vi "72_Vision_RC Servo_DC_Moto_test_PID.vi"() -> ()   [LabVIEW 2018]
uses:
  <userlib>/KNR OS 4.0 LabVIEW Toolkit/Type Definition/Resource.ctl
  <userlib>/KNR OS 4.0 LabVIEW Toolkit/Type Definition/RC Servo Port.ctl
  <userlib>/KNR OS 4.0 LabVIEW Toolkit/Type Definition/DC Motor Port.ctl
panel:
  out "Velocity (cm/sec) chart":dbl(graph)
  out "Velocity (cm/sec)":dbl
  in  "Kd":dbl(slide)=0.047 scale=0.0..0.1
  in  "Ki":dbl(slide)=0.035 scale=0.0..0.1
  in  "Kp":dbl(slide)=0.08 scale=0.0..0.2
  out "Desire Velosity":dbl
  out "area":dbl
  out "RC Pulse Width (uS)":u16[](array[numeric])
  out "Image Out":T1(plugin-control)
  in  "stop":bool
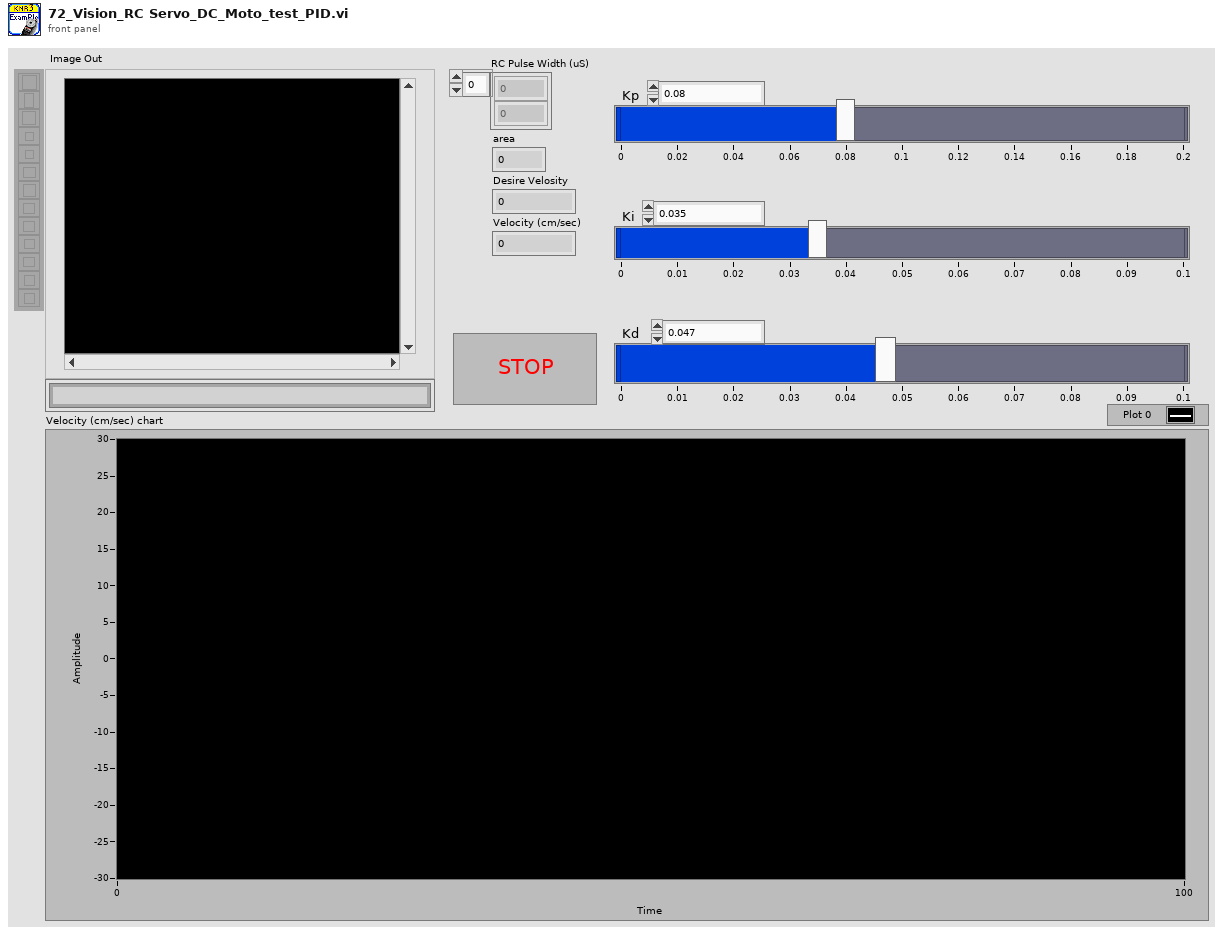
[diagram p1: front panel]
types:
  T1 = typedef "IMAQ Image.ctl" = refnum<image>
  T2 = typedef "RC Servo Port.ctl" = u16
  T3 = typedef "Resource.ctl" = enum16{"KNRm_DDRC", "KNRm_DDDD", "KNRm_DDDR", "KNRm_DDDC", "KNR", "KNRm_neww"}
  T4 = typedef "KNR3 Reference.ctl" = cluster{"FPGA Session":refnum<class "FPGA Interface Base.lvclass">, "Resource":T3}
  T5 = typedef "DC Motor Port.ctl" = u16
  T6 = cluster{"Left":dbl, "Top":dbl, "Right":dbl, "Bottom":dbl}
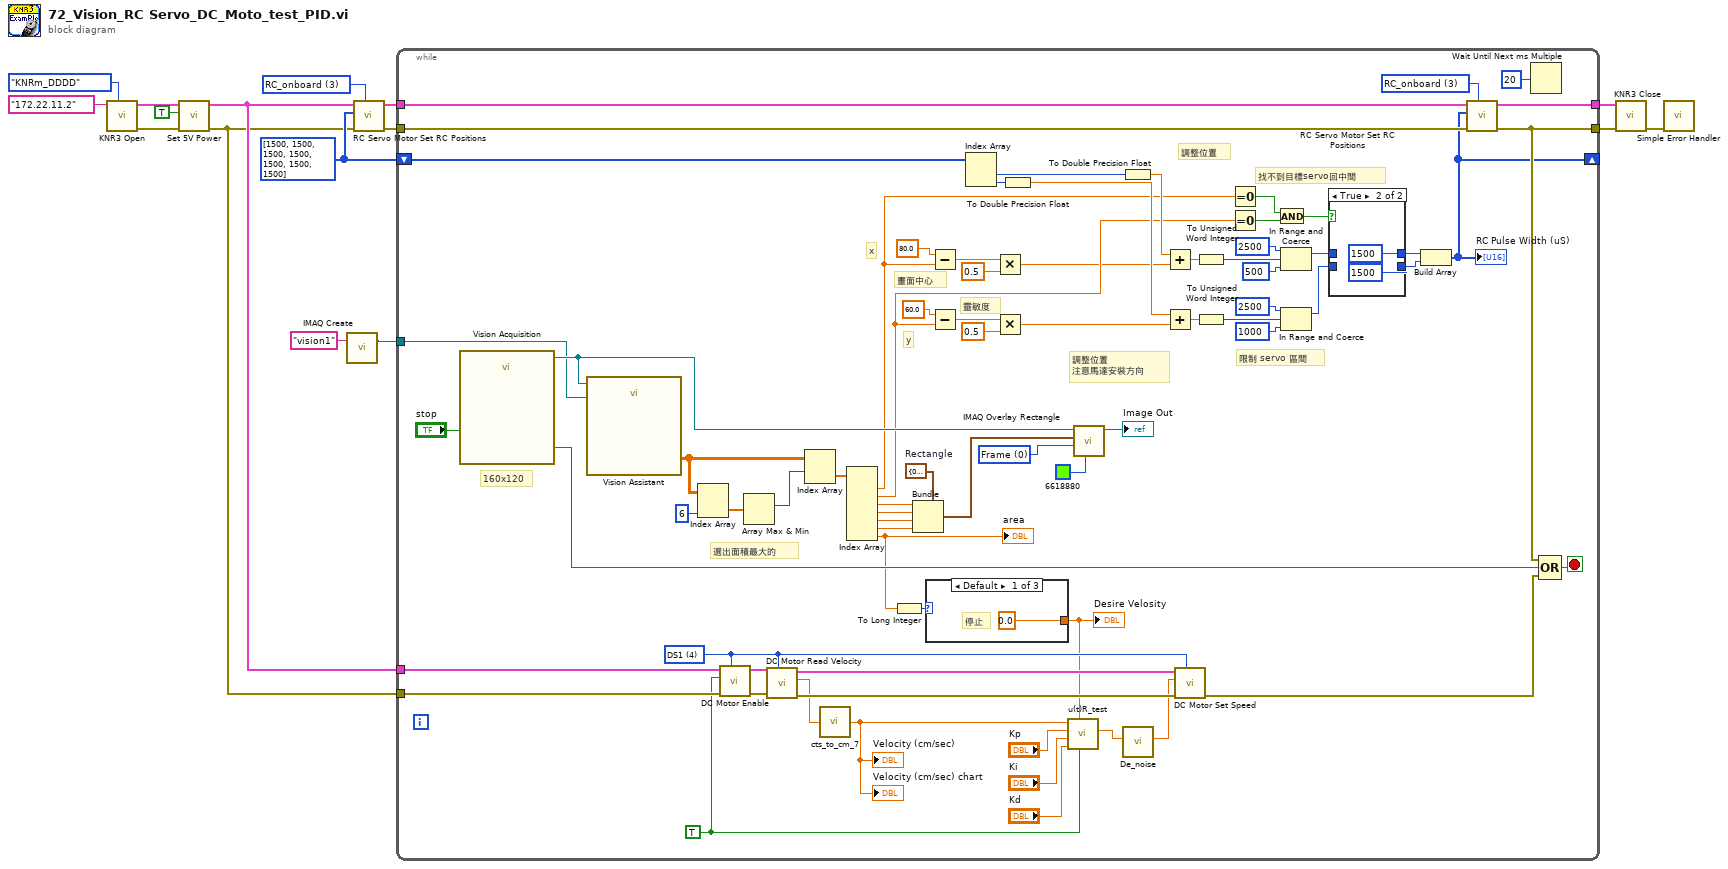
[diagram p0: block diagram]
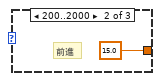
[diagram p2: hidden frame]
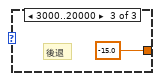
[diagram p3: hidden frame]
diagram:
  w3 = u16[] [1500, 1500, 1500, 1500, 1500, 1500, 1500] ("RC Pulse Width (1500 uS)")
  w6 = T2 3 items=["RC_onboard"=3, "RC_box"=9] ("Port (RC_onboard)")
  n1 = call <userlib>:"KNR3 Open.vi"("Resource"=Resource."KNRm_DDDD", "IP"="172.22.11.2") -> ("error out"=w14:errorcluster, "KNR out"=w15:T4)  [unwired: 8 in]
  n2 = call <userlib>:"Set 5V Power.vi"("error in (no error)"=w14, "5V Power(T)"=TRUE ("5V Power"), "KNR in"=w15) -> ("error out"=w1:errorcluster, "KNR out"=w2:T4)  [unwired: 7 in]
  n3 = call "IMAQ Create"("Image Name"="vision1") -> ("New Image"=w4:T1)  [unwired: 4 in, 1 out]
  n4 = call <userlib>:"RC Servo Motor Set RC Positions.vi"("Port (RC_onboard)"=w6, "RC Pulse Width (1500 uS)"=w3, "KNR in"=w2) -> ("KNR out"=w7:T4)  [unwired: 7 in, 1 out]
  n5 = while {
    tunnel: w7 -> [w90]
    tunnel: [w89] -> w9
    tunnel: w1 -> [w88]
    tunnel: [w86] -> w8
    tunnel: w4 -> [w69]
    shift-right: [w53] -> _
    shift-left: w3 -> [w56]
    tunnel: w2 -> [w26]
    tunnel: w1 -> [w25]
    stop <- w87 stop-if-true
    w24 = u32 0 items=["Frame", "Fill", "Highlight"] ("Drawing Mode (Frame)")
    w19 = TRUE ("Enable Motor(F)")
    w35 = T5 4 items=["DS1"=4, "DS2"=5, "DS3"=6, "DS4"=7] ("Port 2")
    w82 = T6 {"Left"=0.0, "Top"=0.0, "Right"=0.0, "Bottom"=0.0}  # Rectangle
    w84 = T2 3 items=["RC_onboard"=3, "RC_box"=9] ("RC Motor")
    # "調整位置\n注意馬達安裝方向"
    # "調整位置"
    # "畫面中心"
    # "靈敏度"
    # "限制 servo 區間"
    # "找不到目標servo回中間"
    # "y"
    # "x"
    # "160x120"
    # "選出面積最大的"
    n6 = call "Vision Acquisition"("Stop (F)"="stop") -> ("Image Out"=w74:T1, "Stopped"=w67:bool)  [unwired: 24 in, 1 out]
    n7 = call "Vision Assistant"("Image In"=w74, "Image Dst"=w69) -> ("Particle Measurements (Pixels) (Particle Analysis 1)"=w73:dbl[][])  [unwired: 22 in, 3 out]
    n8 = Index Array "Index Array"(array=w73, index (col)=6 ("disabled index (col)")) -> (element=w72:dbl[])  [unwired: 1 in]
    n9 = call <userlib>:"DC Motor Enable.vi"("Port (DS1)"=w35, "error in (no error)"=w25, "Enable Motor(F)"=w19, "KNR in"=w26) -> ("error out"=w31:errorcluster, "KNR out"=w30:T4)  [unwired: 6 in]
    n10 = Array Max & Min(array=w72) -> (max index (indices)=w71:i32)  [unwired: 3 out]
    n11 = call <userlib>:"DC Motor Read Velocity.vi"("Port (DS1)"=w35, "error in (no error)"=w31, "KNR in"=w30) -> ("error out"=w34:errorcluster, "Velocity (cts/sec)"=w32:dbl, "KNR out"=w33:T4)  [unwired: 6 in]
    n12 = Index Array "Index Array"(array=w73, index (row)=w71) -> (element=w83:dbl[])  [unwired: 1 in]
    n13 = call "cts_to_cm_7.vi"("cts"=w32) -> ("cm"=w18:dbl)
    "Velocity (cm/sec)" <- w18
    "Velocity (cm/sec) chart" <- w18
    n14 = Index Array "Index Array"(array=w83) -> (element #1=w46:dbl, element #2=w45:dbl, element #3=w81:dbl, element #4=w80:dbl, element #5=w79:dbl, element #6=w78:dbl, element #7=w28:dbl)  [unwired: 7 in]
    "area" <- w28
    n15 = To Long Integer(number=w28) -> (32bit integer=w23:i32)
    n16 = Bundle "Bundle"(cluster=w82, "Left"=w81, "Top"=w80, "Right"=w79, "Bottom"=w78) -> (w77:T6)
    n17 = case shown="Default" w23 {
      tunnel: [0.0 15.0 -15.0] -> w17
      frame Default {
        # "停止"
      }
      frame 200..2000 {
        # "前進"
      }
      frame 3000..20000 {
        # "後退"
      }
    }
    "Desire Velosity" <- w17
    n18 = Subtract(x=80.0 ("y"), y=w46) -> (x-y=w63:dbl)
    n19 = Subtract(x=60.0 ("y"), y=w45) -> (x-y=w64:dbl)
    n20 = Index Array "Index Array"(array=w56) -> (element #1=w55:u16, element #2=w54:u16)  [unwired: 2 in]
    n21 = Multiply(x=w63, y=0.5) -> (x*y=w44:dbl)
    n22 = Multiply(x=w64, y=0.5) -> (x*y=w43:dbl)
    n23 = To Double Precision Float(number=w54) -> (double precision float=w47:dbl)
    n24 = call "u(t)R_test.vi"("enable"=w19, "Desire Velosity"=w17, "Kd"="Kd", "Ki"="Ki", "Kp"="Kp", "Velocity"=w18) -> ("u(t)"=w29:dbl)  [unwired: 5 in]
    n25 = call "IMAQ Overlay Rectangle"("Color"=u32 6618880, "Drawing Mode (Frame)"=w24, "Rectangle"=w77, "Image"=w74) -> ("Image Out"=→"Image Out":T1)  [unwired: 6 in, 1 out]
    n26 = To Double Precision Float(number=w55) -> (double precision float=w48:dbl)
    n27 = call "De_noise.vi"("u(t)"=w29) -> ("u(t)2"=w16:dbl)  [unwired: 6 in]
    n28 = Add(x=w48, y=w44) -> (x+y=w65:dbl)
    n29 = Add(x=w47, y=w43) -> (x+y=w66:dbl)
    n30 = call <userlib>:"DC Motor Set Speed.vi"("Port (DS1)"=w35, "error in (no error)"=w34, "Speed (+-100%)"=w16, "KNR in"=w33) -> ("error out"=w27:errorcluster)  [unwired: 6 in, 1 out]
    n31 = To Unsigned Word Integer(number=w65) -> (unsigned 16bit integer=w50:u16)
    n32 = To Unsigned Word Integer(number=w66) -> (unsigned 16bit integer=w49:u16)
    n33 = Equal To 0?(x=w46) -> (x = 0?=w40:bool)
    n34 = Equal To 0?(x=w45) -> (x = 0?=w41:bool)
    n35 = And(x=w40, y=w41) -> (x .and. y?=w42:bool)
    n36 = In Range and Coerce(upper limit=u16 2500, x=w50, lower limit=u16 500) -> (coerced(x)=w39:u16)  [unwired: 1 out]
    n37 = In Range and Coerce(upper limit=u16 2500, x=w49, lower limit=u16 1000) -> (coerced(x)=w38:u16)  [unwired: 1 out]
    n38 = case shown="True" w42 {
      tunnel: w39 -> [w95 _]
      tunnel: w38 -> [w94 _]
      tunnel: [w95 u16 1500] -> w37
      tunnel: [w94 u16 1500] -> w36
      frame False {
      }
      frame True {
      }
    }
    n39 = Build Array(w37, w36) -> (w53:u16[])
    "RC Pulse Width (uS)" <- w53
    n40 = call <userlib>:"RC Servo Motor Set RC Positions.vi"("Port (RC_onboard)"=w84, "error in (no error)"=w88, "RC Pulse Width (1500 uS)"=w53, "KNR in"=w90) -> ("error out"=w86:errorcluster, "KNR out"=w89:T4)  [unwired: 6 in]
    n41 = Wait Until Next ms Multiple(millisecond multiple=u32 20) -> ()  [unwired: 1 out]
    n42 = Compound Arithmetic op=OR(w86, w67, w27) -> (w87:bool)
  }
  n43 = call <userlib>:"KNR3 Close.vi"("error in (no error)"=w8, "KNR in"=w9) -> ("error out"=w13:errorcluster)  [unwired: 9 in]
  n44 = call <vilib>:"Simple Error Handler.vi"("error in (no error)"=w13) -> ()  [unwired: 4 in, 5 out]
